vi "Webcam_Open.vi"(7 "webcamnum":i32, 8 "error in (no error)":errorcluster, 10 "height":u32, 11 "width":u32) -> (0 "error out":errorcluster, 3 "return type":i32)   [LabVIEW 2014, in "QwaveSys RPi Training Library.lvlib"]
uses:
  <vilib>/Q-Wave Systems/QwaveSys RPi Training Package (Demo)/Addons/QwaveSys RPi Training Library.lvlib
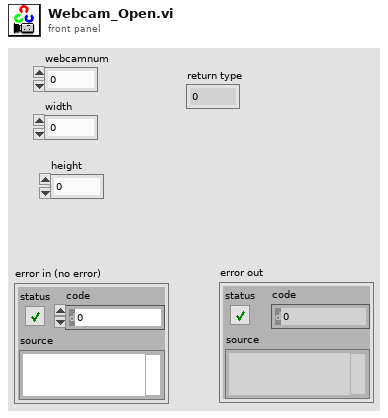
[diagram p1: front panel]
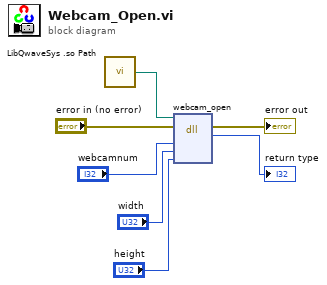
[diagram p0: block diagram]
diagram:
  n1 = call <vilib>:"LibQwaveSys .so Path.vi"() -> ("Lib QwaveSys .so Path"=w1:path)  [unwired: 5 in]
  n2 = dll-call lib="libqwavesys.so" fn="webcam_open"(path in=w1, error in="error in (no error)", "webcamnum"="webcamnum", "width"="width", "height"="height") -> (error out=→"error out":errorcluster, "return type"=→"return type":i32)  [unwired: 4 in, 1 out]
